vi "Compass sim on GIC.vi"(11 "GIC Input":T1={"     Use ?\nOff       On"=[FALSE, TRUE, FALSE, TRUE], "Mode:"=FALSE, "Extra Port"="", "Hokuyo Port"="COM7", "Tx Prop  Port"="COM6", "Compass Port"="", "GPS Port"="", "Num of WPs"=0, "WP Lats and Longs"={"WP Lats"=[], "WP Longs"=[]}, "Obst Lats and Longs"={"Obst Lats"=[], "Obst Longs"=[]}, "Parameters"=[], "GPS Data"=[], "Compass"=0.0, "LMS Vector"=[], "Vision Vector"=[], "Direction Cmd"=0.0, "Speed Cmd"=0.0, "WP Vector"=[], "WP Number"=0, "Extra"=0, "SW Map"=[], "Path Cluster"={"Path x node"=[], "Path y node"=[]}, "Sim Course"=[]} {"Obst Lats and Longs"."Obst Longs" format="%#_8g"; "Obst Lats and Longs"."Obst Lats" format="%#_8g"}) -> (3 "GIC Output":T1={"     Use ?\nOff       On"=[FALSE, TRUE, FALSE, TRUE], "Mode:"=FALSE, "Extra Port"="", "Hokuyo Port"="COM7", "Tx Prop  Port"="COM6", "Compass Port"="", "GPS Port"="", "Num of WPs"=0, "WP Lats and Longs"={"WP Lats"=[], "WP Longs"=[]}, "Obst Lats and Longs"={"Obst Lats"=[], "Obst Longs"=[]}, "Parameters"=[], "GPS Data"=[], "Compass"=0.0, "LMS Vector"=[], "Vision Vector"=[], "Direction Cmd"=0.0, "Speed Cmd"=0.0, "WP Vector"=[], "WP Number"=0, "Extra"=0, "SW Map"=[], "Path Cluster"={"Path x node"=[], "Path y node"=[]}, "Sim Course"=[]} {"Obst Lats and Longs"."Obst Longs" format="%#_8g"; "Obst Lats and Longs"."Obst Lats" format="%#_8g"})   [LabVIEW 2014]
uses:
  Global_vars.vi
panel:
  out "compass out":dbl
  # "Compass sim on  GIC"
  # "Input:"
  # "Output:"
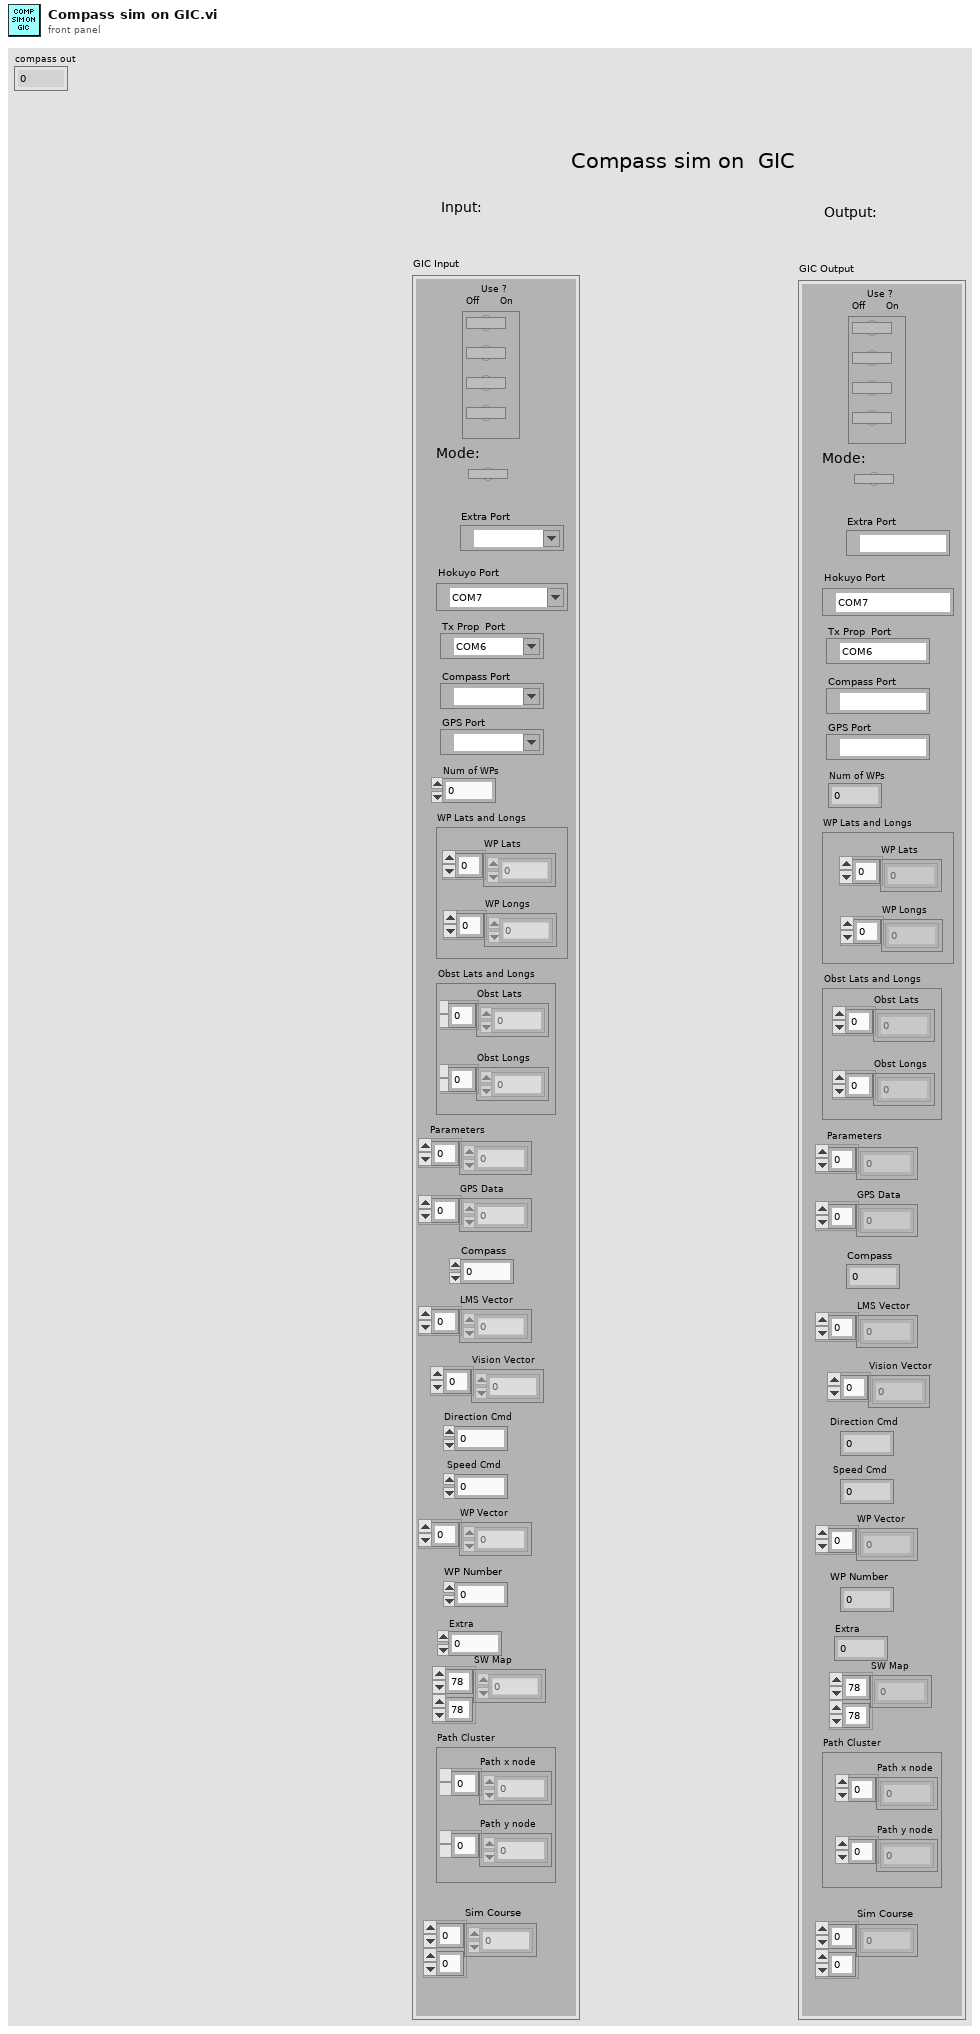
[diagram p1: front panel]
types:
  T1 = cluster{"     Use ?\nOff       On":bool[], "Mode:":bool, "Extra Port":refnum<visa-resource-name>, "Hokuyo Port":refnum<visa-resource-name>, "Tx Prop  Port":refnum<visa-resource-name>, "Compass Port":refnum<visa-resource-name>, "GPS Port":refnum<visa-resource-name>, "Num of WPs":i16, "WP Lats and Longs":cluster{"WP Lats":dbl[], "WP Longs":dbl[]}, "Obst Lats and Longs":cluster{"Obst Lats":dbl[], "Obst Longs":dbl[]}, "Parameters":dbl[], "GPS Data":dbl[], "Compass":dbl, "LMS Vector":dbl[], "Vision Vector":dbl[], "Direction Cmd":dbl, "Speed Cmd":dbl, "WP Vector":dbl[], "WP Number":i32, "Extra":i16, "SW Map":i32[][], "Path Cluster":cluster{"Path x node":dbl[], "Path y node":dbl[]}, "Sim Course":i8[][]}
  T2 = cluster{"     Use ?\nOff       On":bool[], "Mode:":bool, "Rx Prop Port":refnum<visa-resource-name>, "Hokuyo Port":refnum<visa-resource-name>, "Tx Prop  Port":refnum<visa-resource-name>, "Compass Port":refnum<visa-resource-name>, "GPS Port":refnum<visa-resource-name>, "Num of WPs":i16, "WP Lats and Longs":cluster{"WP Lats":dbl[], "WP Longs":dbl[]}, "Obst Lats and Longs":cluster{"Obst Lats":dbl[], "Obst Longs":dbl[]}, "Parameters":dbl[], "GPS Data":dbl[], "Compass":dbl, "LMS Vector":dbl[], "Vision Vector":dbl[], "Direction Cmd":dbl, "Speed Cmd":dbl, "WP Vector":dbl[], "WP Number":i32, "Extra":i16, "SW Map":i32[][], "Path Cluster":cluster{"Path x node":dbl[], "Path y node":dbl[]}, "Sim Course":i8[][]}
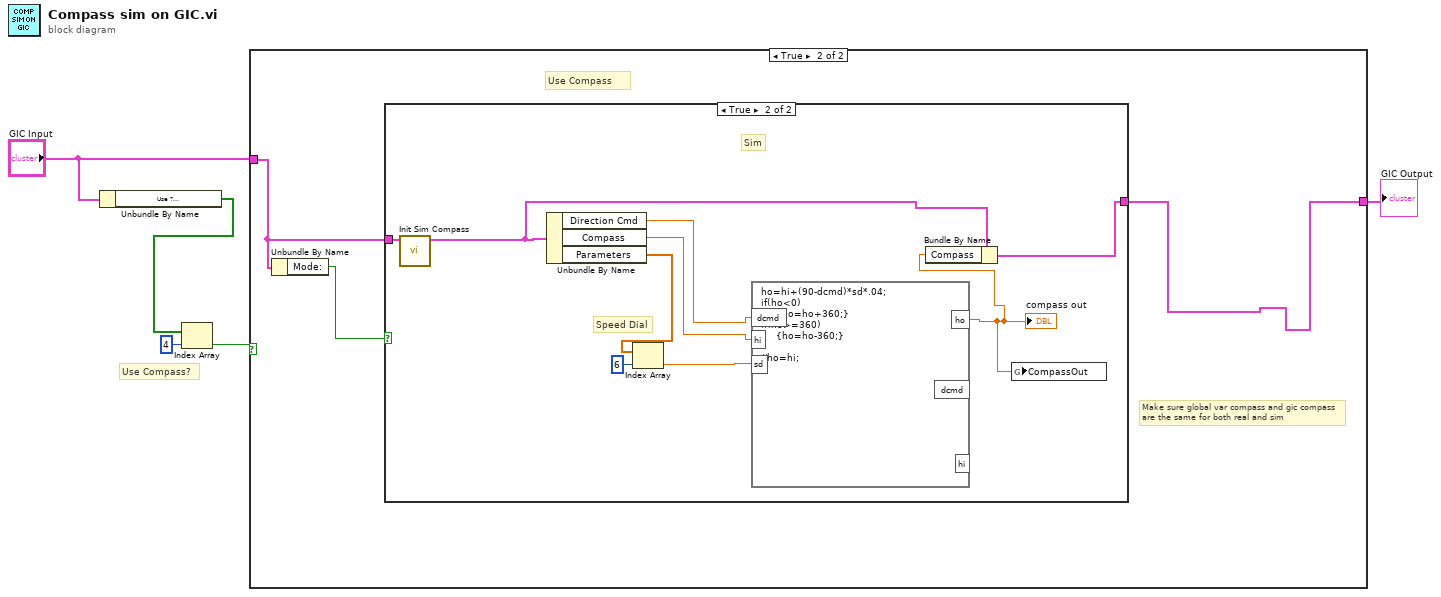
[diagram p0: block diagram]
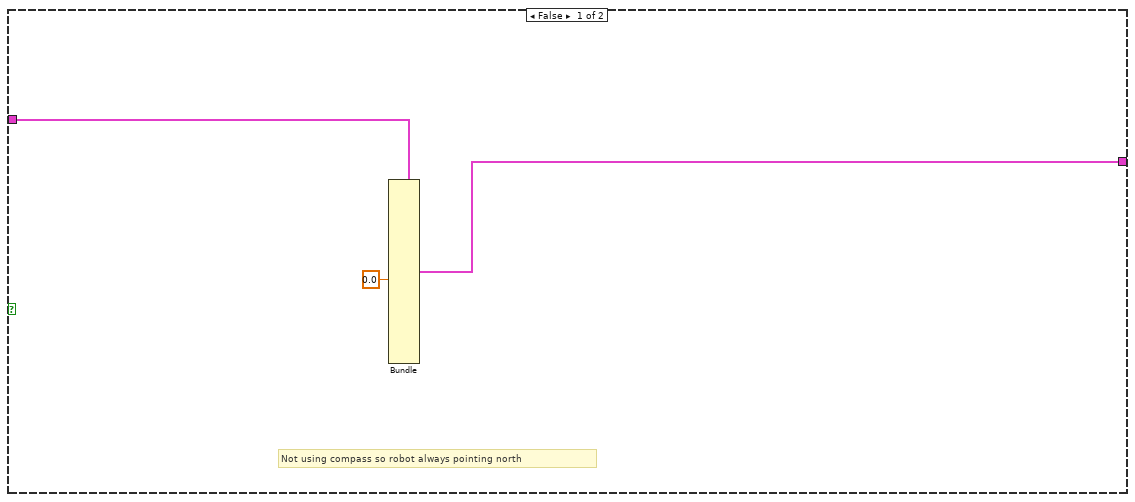
[diagram p2: hidden frame]
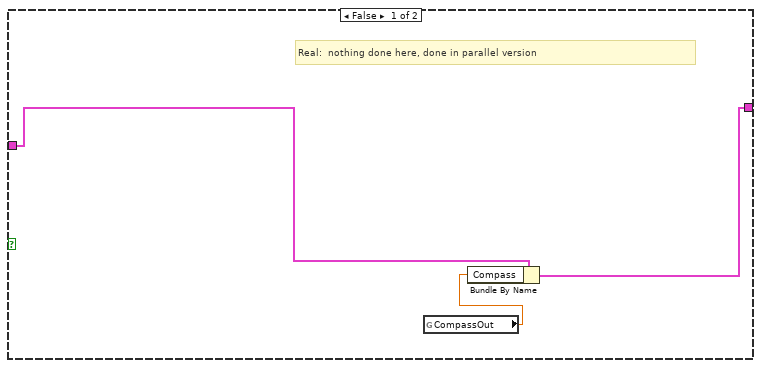
[diagram p3: hidden frame]
diagram:
  # "Use Compass?"
  n1 = Unbundle By Name("GIC Input") -> ("Use ?\nOff       On"=w5:bool[])
  n2 = Index Array(array=w5, index=4) -> (element=w3:bool)
  n3 = case shown="True" w3 {
    tunnel: "GIC Input" -> [w8 w11]
    tunnel: [w6 w9] -> w1
    frame False {
      # "Not using compass so robot always pointing north"
      n4 = Bundle(cluster=w8, "Compass"=0.0) -> (w6:T1)  [unwired: 22 in]
    }
    frame True {
      # "Make sure global var compass and gic compass\nare the same for both real and sim"
      # "Use Compass"
      n5 = Unbundle By Name(w11) -> ("Mode:"=w10:bool)
      n6 = case shown="True" w10 {
        tunnel: w11 -> [w14 w18]
        tunnel: [w12 w15] -> w9
        frame False {
          # "Real:  nothing done here, done in parallel version"
          n7 = global read "Global_vars.vi" "CompassOut"() -> (w13:dbl)
          n8 = Bundle By Name(cluster=w14, "Compass"=w13) -> (w12:T1)
        }
        frame True {
          # "Sim"
          # "Speed Dial"
          n9 = call "Init Sim Compass.vi"("GIC Input"=w18) -> ("GIC Output"=w17:T2)  [unwired: 10 in]
          n10 = Unbundle By Name(w17) -> ("Direction Cmd"=w20:dbl, "Compass"=w19:dbl, "Parameters"=w23:dbl[])
          n11 = Index Array(array=w23, index=6) -> (element=w21:dbl)
          n12 = formula code="ho=hi+(90-dcmd)*sd*.04;\nif(ho<0)\n     {ho=ho+360;}\nif(ho>=360)\n     {ho=ho-360;}\n\n//ho=hi;"("dcmd"=w20, "hi"=w19, "sd"=w21) -> ("ho"=w16:dbl)  [unwired: 2 out]
          "compass out" <- w16
          n13 = Bundle By Name(cluster=w17, "Compass"=w16) -> (w15:T2)
          n14 = global write "Global_vars.vi" "CompassOut"(w16) -> ()
        }
      }
    }
  }
  "GIC Output" <- w1
